vi "T1T2占空比.vi"() -> ()   [LabVIEW 2019]
uses:
  <vilib>/DAQmx/read.llb/DAQmx Read (Counter 1D DBL 1Chan NSamp).vi
  Global_Variable/Global.vi
  <vilib>/DAQmx/create/channels.llb/DAQmx Create Channel (CI-Period).vi
  <vilib>/DAQmx/configure/timing.llb/DAQmx Timing (Implicit).vi
  <vilib>/DAQmx/miscellaneous.llb/DAQmx Fill In Error Info.vi
  <userlib>/_MGI/1D Array/MGI Average/MGI Average (DBL[]).vi
  <vilib>/DAQmx/create/channels.llb/DAQmx Create Channel (CI-Pulse Width).vi
  <resource>/objmgr/daqmx.rc
panel:
  out "T2":dbl
  out "T2周期":dbl
  out "T1周期":dbl
  out "T1":dbl
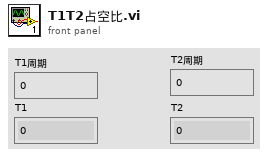
[diagram p1: front panel]
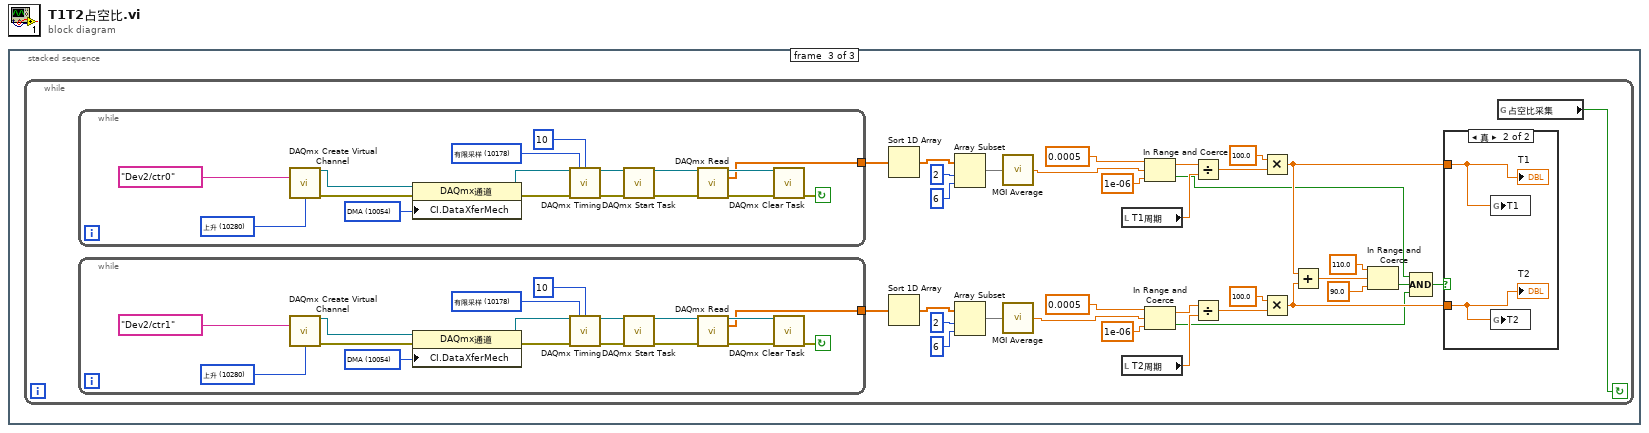
[diagram p0: block diagram]
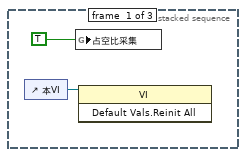
[diagram p2: hidden frame]
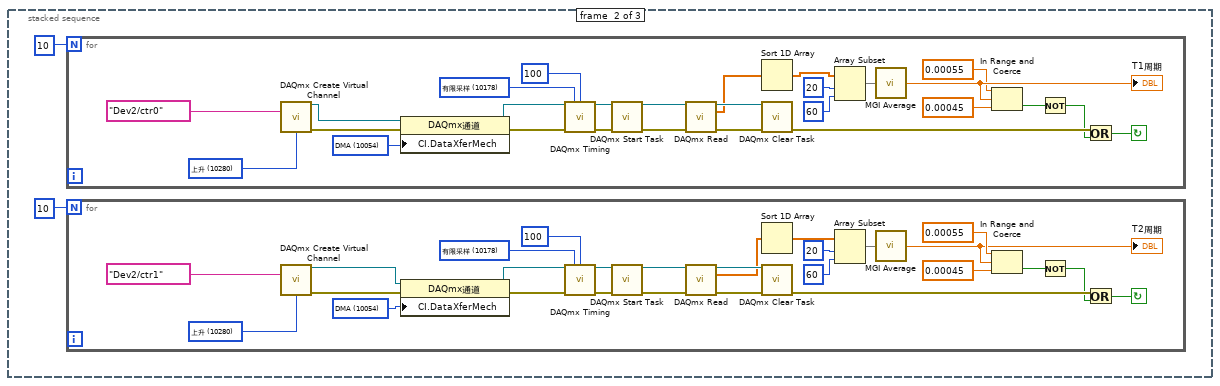
[diagram p3: hidden frame]
diagram:
  n1 = stacked-sequence {
    frame #0 {
      n2 = control-ref of="本VI"() -> (w2:refnum<vi>)
      n3 = global write "Global.vi" "占空比采集"(TRUE ("工位一占空比采集")) -> ()
      n4 = invoke class="VI" method="Default Vals.Reinit All"(reference=w2) -> ()  [unwired: 2 in, 3 out]
    }
    frame #1 {
      n5 = for {
        N: 10 -> [_]
        stop <- w32 continue-if-true
        w45 = 10054 items=["DMA"=10054, "中断"=10204, "程序控制I/O"=10264, "USB Bulk"=12590] ("CI.DataXferMech")
        w49 = 10178 items=["有限采样"=10178, "连续采样"=10123, "硬件定时单点"=12522] ("sample mode")
        w58 = 10280 items=["上升"=10280, "下降"=10171] ("starting edge")
        n6 = call-poly <vilib>:"DAQmx Create Virtual Channel.vi"("counter"=tag "Dev2/ctr0", "starting edge"=w58) -> ("task out"=w57:refnum<k21>, "error out"=w47:errorcluster)  [unwired: 12 in]
        n7 = property class="DAQmx通道"(reference=w57, error in=w47, "CI.DataXferMech"=w45) -> (reference out=w48:refnum<k21>, error out=w46:errorcluster)
        n8 = call-poly <vilib>:"DAQmx Timing.vi"("task/channels in"=w48, "sample mode"=w49, "samples per channel"=100, "error in"=w46) -> ("task out"=w56:refnum<k21>, "error out"=w55:errorcluster)  [unwired: 10 in]
        n9 = call <vilib>:"DAQmx Start Task.vi"("task/channels in"=w56, "error in"=w55) -> ("task out"=w54:refnum<k21>, "error out"=w53:errorcluster)  [unwired: 12 in]
        n10 = call-poly <vilib>:"DAQmx Read.vi"("task/channels in"=w54, "error in"=w53) -> ("task out"=w51:refnum<k21>, "data"=w39:dbl[], "error out"=w52:errorcluster)  [unwired: 11 in]
        n11 = Sort 1D Array(array=w39) -> (sorted array=w42:dbl[])
        n12 = call <vilib>:"DAQmx Clear Task.vi"("task in"=w51, "error in"=w52) -> ("error out"=w34:errorcluster)  [unwired: 13 in]
        n13 = Array Subset(array=w42, index=20 ("索引"), length=60 ("长度")) -> (w43:dbl[])
        n14 = call-poly <userlib>:"MGI Average.vi"("Double[]"=w43) -> ("Average"=w38:dbl)  [unwired: 1 in]
        "T1周期" <- w38
        n15 = In Range and Coerce(upper limit=0.00055 ("上限"), x=w38, lower limit=0.00045 ("上限")) -> (In Range?=w35:bool)  [unwired: 1 out]
        n16 = Not(x=w35) -> (.not. x?=w33:bool)
        n17 = Or(x=w34, y=w33) -> (x .or. y?=w32:bool)
      }
      n18 = for {
        N: 10 -> [_]
        stop <- w5 continue-if-true
        w18 = 10054 items=["DMA"=10054, "中断"=10204, "程序控制I/O"=10264, "USB Bulk"=12590] ("CI.DataXferMech")
        w22 = 10178 items=["有限采样"=10178, "连续采样"=10123, "硬件定时单点"=12522] ("sample mode")
        w31 = 10280 items=["上升"=10280, "下降"=10171] ("starting edge")
        n19 = call-poly <vilib>:"DAQmx Create Virtual Channel.vi"("counter"=tag "Dev2/ctr1", "starting edge"=w31) -> ("task out"=w30:refnum<k21>, "error out"=w20:errorcluster)  [unwired: 12 in]
        n20 = property class="DAQmx通道"(reference=w30, error in=w20, "CI.DataXferMech"=w18) -> (reference out=w21:refnum<k21>, error out=w19:errorcluster)
        n21 = call-poly <vilib>:"DAQmx Timing.vi"("task/channels in"=w21, "sample mode"=w22, "samples per channel"=100, "error in"=w19) -> ("task out"=w29:refnum<k21>, "error out"=w28:errorcluster)  [unwired: 10 in]
        n22 = call <vilib>:"DAQmx Start Task.vi"("task/channels in"=w29, "error in"=w28) -> ("task out"=w27:refnum<k21>, "error out"=w26:errorcluster)  [unwired: 12 in]
        n23 = call-poly <vilib>:"DAQmx Read.vi"("task/channels in"=w27, "error in"=w26) -> ("task out"=w24:refnum<k21>, "data"=w12:dbl[], "error out"=w25:errorcluster)  [unwired: 11 in]
        n24 = Sort 1D Array(array=w12) -> (sorted array=w16:dbl[])
        n25 = call <vilib>:"DAQmx Clear Task.vi"("task in"=w24, "error in"=w25) -> ("error out"=w8:errorcluster)  [unwired: 13 in]
        n26 = Array Subset(array=w16, index=20 ("索引"), length=60 ("长度")) -> (w15:dbl[])
        n27 = call-poly <userlib>:"MGI Average.vi"("Double[]"=w15) -> ("Average"=w9:dbl)  [unwired: 1 in]
        "T2周期" <- w9
        n28 = In Range and Coerce(upper limit=0.00055 ("上限"), x=w9, lower limit=0.00045 ("上限")) -> (In Range?=w7:bool)  [unwired: 1 out]
        n29 = Not(x=w7) -> (.not. x?=w6:bool)
        n30 = Or(x=w8, y=w6) -> (x .or. y?=w5:bool)
      }
    }
    frame #2 {
      n31 = while {
        stop <- w74 continue-if-true
        n32 = while {
          tunnel: [w118] -> w92
          stop <- w112 continue-if-true
          w114 = 10054 items=["DMA"=10054, "中断"=10204, "程序控制I/O"=10264, "USB Bulk"=12590] ("CI.DataXferMech")
          w119 = 10178 items=["有限采样"=10178, "连续采样"=10123, "硬件定时单点"=12522] ("sample mode")
          w128 = 10280 items=["上升"=10280, "下降"=10171] ("starting edge")
          n33 = call-poly <vilib>:"DAQmx Create Virtual Channel.vi"("counter"=tag "Dev2/ctr0", "starting edge"=w128) -> ("task out"=w127:refnum<k21>, "error out"=w116:errorcluster)  [unwired: 12 in]
          n34 = property class="DAQmx通道"(reference=w127, error in=w116, "CI.DataXferMech"=w114) -> (reference out=w117:refnum<k21>, error out=w115:errorcluster)
          n35 = call-poly <vilib>:"DAQmx Timing.vi"("task/channels in"=w117, "sample mode"=w119, "samples per channel"=10, "error in"=w115) -> ("task out"=w126:refnum<k21>, "error out"=w125:errorcluster)  [unwired: 10 in]
          n36 = call <vilib>:"DAQmx Start Task.vi"("task/channels in"=w126, "error in"=w125) -> ("task out"=w124:refnum<k21>, "error out"=w123:errorcluster)  [unwired: 12 in]
          n37 = call-poly <vilib>:"DAQmx Read.vi"("task/channels in"=w124, "error in"=w123) -> ("task out"=w121:refnum<k21>, "data"=w118:dbl[], "error out"=w122:errorcluster)  [unwired: 11 in]
          n38 = call <vilib>:"DAQmx Clear Task.vi"("task in"=w121, "error in"=w122) -> ("error out"=w112:errorcluster)  [unwired: 13 in]
        }
        n39 = while {
          tunnel: [w101] -> w87
          stop <- w95 continue-if-true
          w97 = 10054 items=["DMA"=10054, "中断"=10204, "程序控制I/O"=10264, "USB Bulk"=12590] ("CI.DataXferMech")
          w102 = 10178 items=["有限采样"=10178, "连续采样"=10123, "硬件定时单点"=12522] ("sample mode")
          w111 = 10280 items=["上升"=10280, "下降"=10171] ("starting edge")
          n40 = call-poly <vilib>:"DAQmx Create Virtual Channel.vi"("counter"=tag "Dev2/ctr1", "starting edge"=w111) -> ("task out"=w110:refnum<k21>, "error out"=w99:errorcluster)  [unwired: 12 in]
          n41 = property class="DAQmx通道"(reference=w110, error in=w99, "CI.DataXferMech"=w97) -> (reference out=w100:refnum<k21>, error out=w98:errorcluster)
          n42 = call-poly <vilib>:"DAQmx Timing.vi"("task/channels in"=w100, "sample mode"=w102, "samples per channel"=10, "error in"=w98) -> ("task out"=w109:refnum<k21>, "error out"=w108:errorcluster)  [unwired: 10 in]
          n43 = call <vilib>:"DAQmx Start Task.vi"("task/channels in"=w109, "error in"=w108) -> ("task out"=w107:refnum<k21>, "error out"=w106:errorcluster)  [unwired: 12 in]
          n44 = call-poly <vilib>:"DAQmx Read.vi"("task/channels in"=w107, "error in"=w106) -> ("task out"=w104:refnum<k21>, "data"=w101:dbl[], "error out"=w105:errorcluster)  [unwired: 11 in]
          n45 = call <vilib>:"DAQmx Clear Task.vi"("task in"=w104, "error in"=w105) -> ("error out"=w95:errorcluster)  [unwired: 13 in]
        }
        n46 = Sort 1D Array(array=w92) -> (sorted array=w91:dbl[])
        n47 = Sort 1D Array(array=w87) -> (sorted array=w88:dbl[])
        n48 = Array Subset(array=w91, index=2 ("索引"), length=6 ("长度")) -> (w90:dbl[])
        n49 = Array Subset(array=w88, index=2 ("索引"), length=6 ("长度")) -> (w89:dbl[])
        n50 = call-poly <userlib>:"MGI Average.vi"("Double[]"=w90) -> ("Average"=w82:dbl)  [unwired: 1 in]
        n51 = call-poly <userlib>:"MGI Average.vi"("Double[]"=w89) -> ("Average"=w80:dbl)  [unwired: 1 in]
        n52 = local read "T1周期"() -> (w72:dbl)
        n53 = local read "T2周期"() -> (w70:dbl)
        n54 = In Range and Coerce(upper limit=0.0005 ("上限"), x=w82, lower limit=1e-06 ("上限")) -> (coerced(x)=w81:dbl, In Range?=w62:bool)
        n55 = In Range and Coerce(upper limit=0.0005 ("上限"), x=w80, lower limit=1e-06 ("上限")) -> (coerced(x)=w79:dbl, In Range?=w61:bool)
        n56 = Divide(x=w81, y=w72) -> (x/y=w73:dbl)
        n57 = Divide(x=w79, y=w70) -> (x/y=w69:dbl)
        n58 = Multiply(x=100.0, y=w73) -> (x*y=w67:dbl)
        n59 = Multiply(x=100.0, y=w69) -> (x*y=w66:dbl)
        n60 = Add(x=w67, y=w66) -> (x+y=w65:dbl)
        n61 = In Range and Coerce(upper limit=110.0 ("上限"), x=w65, lower limit=90.0 ("下限")) -> (In Range?=w60:bool)  [unwired: 1 out]
        n62 = Compound Arithmetic op=AND ("复合运算")(w62, w60, w61) -> (w59:bool)
        n63 = case shown="真" w59 {
          tunnel: w67 -> [_ w94]
          tunnel: w66 -> [_ w93]
          frame False {
          }
          frame True {
            n64 = global write "Global.vi" "T1"(w94) -> ()
            n65 = global write "Global.vi" "T2"(w93) -> ()
            "T1" <- w94
            "T2" <- w93
          }
        }
        n66 = global read "Global.vi" "占空比采集"() -> (w74:bool)
      }
    }
  }
